vi "COMI Goto URL.vi"(10 "bMaximize":i32, 11 "szUrl":string) -> ()   [LabVIEW 2017, in "Comidll.lvlib"]
doc: "void (COMI_GotoURL) (const char *szUrl, int bMaximize);"
uses:
  <userlib>/Comidll/Comidll.lvlib
  <userlib>/Comidll/Comidll.dll
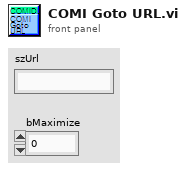
[diagram p1: front panel]
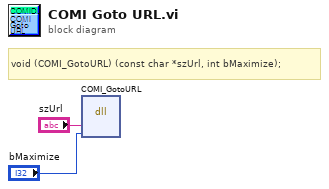
[diagram p0: block diagram]
diagram:
  # "void\t(COMI_GotoURL) (const char *szUrl, int bMaximize);"
  n1 = dll-call lib="C:/Program Files/National Instruments/LabVIEW 2017/user.lib/Comidll/Comidll.*" fn="COMI_GotoURL"("szUrl"="szUrl", "bMaximize"="bMaximize") -> ()  [unwired: 6 in, 2 out]
